vi "logout.vi"(7 "httpRequestID":u32) -> ()   [LabVIEW 2011]
doc: "This VI is a state machine that can be ran from a Browser."
uses:
  server/database/Users/User Record.ctl
  <vilib>/addons/internet/utils/strutil.llb/Case Matching.ctl
  <vilib>/wsapi/subVIs/Write Single Session Variable.vi
  <vilib>/wsapi/NI_WebServices.lvlib
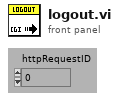
[diagram p1: front panel]
types:
  T1 = typedef "Case Matching.ctl" = enum16{"a != A", "a == A", "system"}
  T2 = typedef "User Record.ctl" = cluster{"ixUser":i32, "sxUsername":string, "sLastName":string, "sFirstName":string, "sEmail":string, "sPassword":string, "tLoginTime":timestamp, "sLoginComputer":string, "fAdministrator":bool, "fRunSequences":bool, "fModifySequences":bool, "fRunScenarios":bool, "fModifyScenarios":bool, "fModifyTemplates":bool, "fModifyUsers":bool, "fModifyStations":bool, "fModifyFields":bool}
  T3 = typedef "Keyed Array.ctl" = cluster{"keys":string[], "values":string[]}
  T4 = typedef "Connection Refnum.ctl" = cluster{"Environment Handle":i32, "Connection Handle":i32}
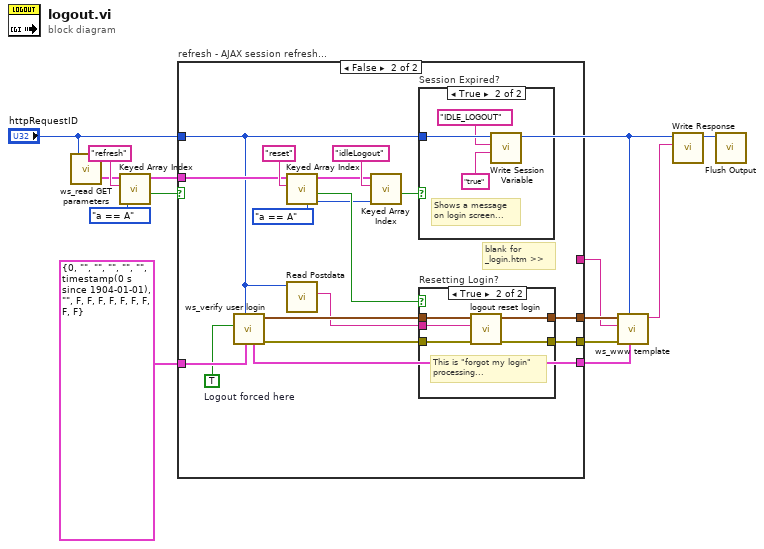
[diagram p0: block diagram]
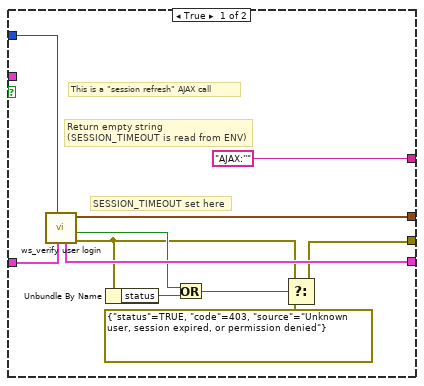
[diagram p2: hidden frame]
diagram:
  n1 = call "ws_read GET parameters.vi"("httpRequestID"="httpRequestID") -> ("GET query params"=w10:T3)  [unwired: 2 in]
  n2 = call <vilib>:"Keyed Array Index.vi"("case matching (sensitive)"=Case_Matching."a == A", "key"="refresh" ("Template (\"\")"), "array in"=w10) -> ("valid key"=w8:bool, "duplicate array"=w9:T3)  [unwired: 1 in, 2 out]
  n3 = case "refresh - AJAX session refresh..." shown="False" w8 {
    tunnel: [w20 w33] -> w6
    tunnel: [w23 w25] -> w7
    tunnel: [w21 w30] -> w1
    tunnel: T2 {"ixUser"=0, "sxUsername"="", "sLastName"="", "sFirstName"="", "sEmail"="", "sPassword"="", "tLoginTime"=timestamp(0 s since 1904-01-01), "sLoginComputer"="", "fAdministrator"=FALSE, "fRunSequences"=FALSE, "fModifySequences"=FALSE, "fRunScenarios"=FALSE, "fModifyScenarios"=FALSE, "fModifyTemplates"=FALSE, "fModifyUsers"=FALSE, "fModifyStations"=FALSE, "fModifyFields"=FALSE} ("Required Permisions") -> [w24 w31]
    tunnel: ["AJAX:''" ("format string") _] -> w2
    tunnel: w9 -> [_ w37]
    tunnel: "httpRequestID" -> [w14 w27]
    frame True {
      # "SESSION_TIMEOUT set here"
      # "Return empty string\n(SESSION_TIMEOUT is read from ENV)"
      # "This is a \"session refresh\" AJAX call"
      n4 = call "ws_verify user login.vi"("Required Permisions"=w24, "httpRequestID"=w14) -> ("error out"=w18:errorcluster, "User Verified\nand Spartan\nAuthorized?"=w19:bool, "DB Connection Ref"=w23:T4, "User"=w21:T2)  [unwired: 6 in]
      n5 = Unbundle By Name(w18) -> ("status"=w17:bool)
      n6 = Or(x=w19, y=w17) -> (x .or. y?=w16:bool)
      n7 = Select(t=w18, s=w16, f=errorcluster {"status"=TRUE, "code"=403, "source"="Unknown user, session expired, or permission denied"}) -> (s? t:f=w20:errorcluster)
    }
    frame False {
      w34 = Case_Matching."a == A" ("case matching (sensitive)")
      w29 = TRUE  # Logout forced here
      # "blank for\n_login.htm >>"
      n8 = call "ws_verify user login.vi"("Required Permisions"=w31, "httpRequestID"=w27, "Logout? (f)"=w29) -> ("error out"=w32:errorcluster, "DB Connection Ref"=w28:T4, "User"=w30:T2)  [unwired: 5 in, 1 out]
      n9 = call <vilib>:"Keyed Array Index.vi"("case matching (sensitive)"=w34, "key"="reset" ("Template (\"\")"), "array in"=w37) -> ("valid key"=w39:bool, "duplicate array"=w36:T3)  [unwired: 1 in, 2 out]
      n10 = call <vilib>:"Read Postdata.vi"("httpRequestID"=w27) -> ("postdata"=w26:string)  [unwired: 8 in, 2 out]
      n11 = call <vilib>:"Keyed Array Index.vi"("case matching (sensitive)"=w34, "key"="idleLogout" ("Template (\"\")"), "array in"=w36) -> ("valid key"=w35:bool)  [unwired: 1 in, 3 out]
      n12 = case "Session Expired?" shown="True" w35 {
        tunnel: w27 -> [_ w42]
        frame False {
        }
        frame True {
          # "Shows a message\non login screen..."
          n13 = call-poly <vilib>:"Write Session Variable.vi"("value"="true", "key"="IDLE_LOGOUT" ("name"), "httpRequestID"=w42) -> ()  [unwired: 5 in, 4 out]
        }
      }
      n14 = case "Resetting Login?" shown="True" w39 {
        tunnel: w26 -> [_ w46]
        tunnel: [w44 w48] -> w25
        tunnel: [w45 w50] -> w33
        tunnel: w32 -> [w45 w49]
        tunnel: w28 -> [w44 w47]
        frame False {
        }
        frame True {
          # "This is \"forgot my login\"\nprocessing..."
          n15 = call "logout reset login.vi"("error in (no error)"=w49, "POST Data (\"\")"=w46, "Connection Refnum"=w47) -> ("error out"=w50:errorcluster, "dup Connection Refnum"=w48:T4)  [unwired: 3 out]
        }
      }
    }
  }
  n16 = call "ws_www template.vi"("User"=w1, "httpRequestID"="httpRequestID", "error in (no error)"=w6, "Template (\"\")"=w2, "DB Connection Ref"=w7) -> ("HTTP Template Content"=w4:string)  [unwired: 6 in]
  n17 = call <vilib>:"Write Response.vi"("response string"=w4, "httpRequestID"="httpRequestID") -> ("httpRequestID out"=w5:u32)  [unwired: 8 in, 1 out]
  n18 = call <vilib>:"Flush Output.vi"("httpRequestID"=w5) -> ()  [unwired: 9 in, 2 out]
